vi "Raycaster_CalcObjectDistance.vi"(10 "Location Info":T1, 11 "Decorations In":T5) -> (3 "Decorations Out":T5)   [LabVIEW 2020]
uses:
  Controls/Map_Objects.ctl
  Controls/Map_Object.ctl
  Controls/Map_Position.ctl
  Controls/Game_State.ctl
  Controls/Player_LocationInfo.ctl
  Controls/Player_LocationInfoAxis.ctl
  Globals/FGV_TileVisibleEnum.ctl
  Map_GetMaps.vi
  <vilib>/Utility/file.llb/Application Directory.vi
  <vilib>/rvi/DataTransferAndStorage/Container/XNode/niFpgaContainer.xnode
  <vilib>/rvi/Memory/Memory_Emulation/nirvimemoryFastEmulation.vi
  <vilib>/rvi/Memory/Memory_Emulation/nirvimemoryEmulation.vi
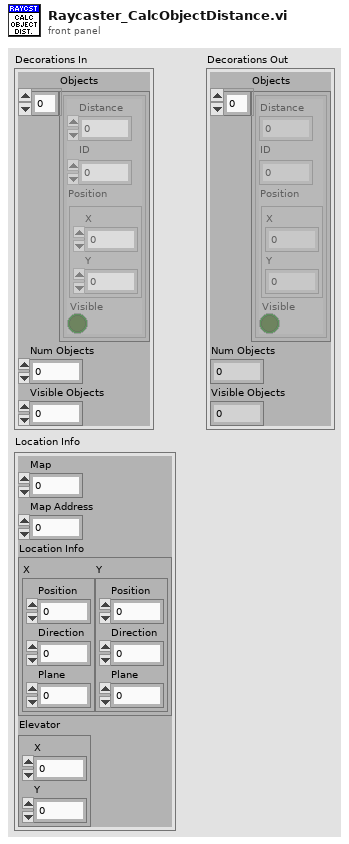
[diagram p1: front panel]
types:
  T1 = typedef "Game_State.ctl" = cluster{"Map":u8, "Map Address":u32, "Location Info":T2, "Elevator":T4}
  T2 = typedef "Player_LocationInfo.ctl" = cluster{"X":T3, "Y":T3}
  T3 = typedef "Player_LocationInfoAxis.ctl" = cluster{"Position":fxp<+/-,32,16>, "Direction":fxp<+/-,32,16>, "Plane":fxp<+/-,32,16>}
  T4 = typedef "Map_Position.ctl" = cluster{"X":fxp<+/-,32,16>, "Y":fxp<+/-,32,16>}
  T5 = typedef "Map_Objects.ctl" = cluster{"Objects":T6[], "Num Objects":i16, "Visible Objects":i16}
  T6 = typedef "Map_Object.ctl" = cluster{"Distance":fxp<+/-,32,16>, "ID":u8, "Position":T4, "Visible":bool}
  T7 = typedef "FGV_TileVisibleEnum.ctl" = enum16{"Reset", "Set Value", "Read Value"}
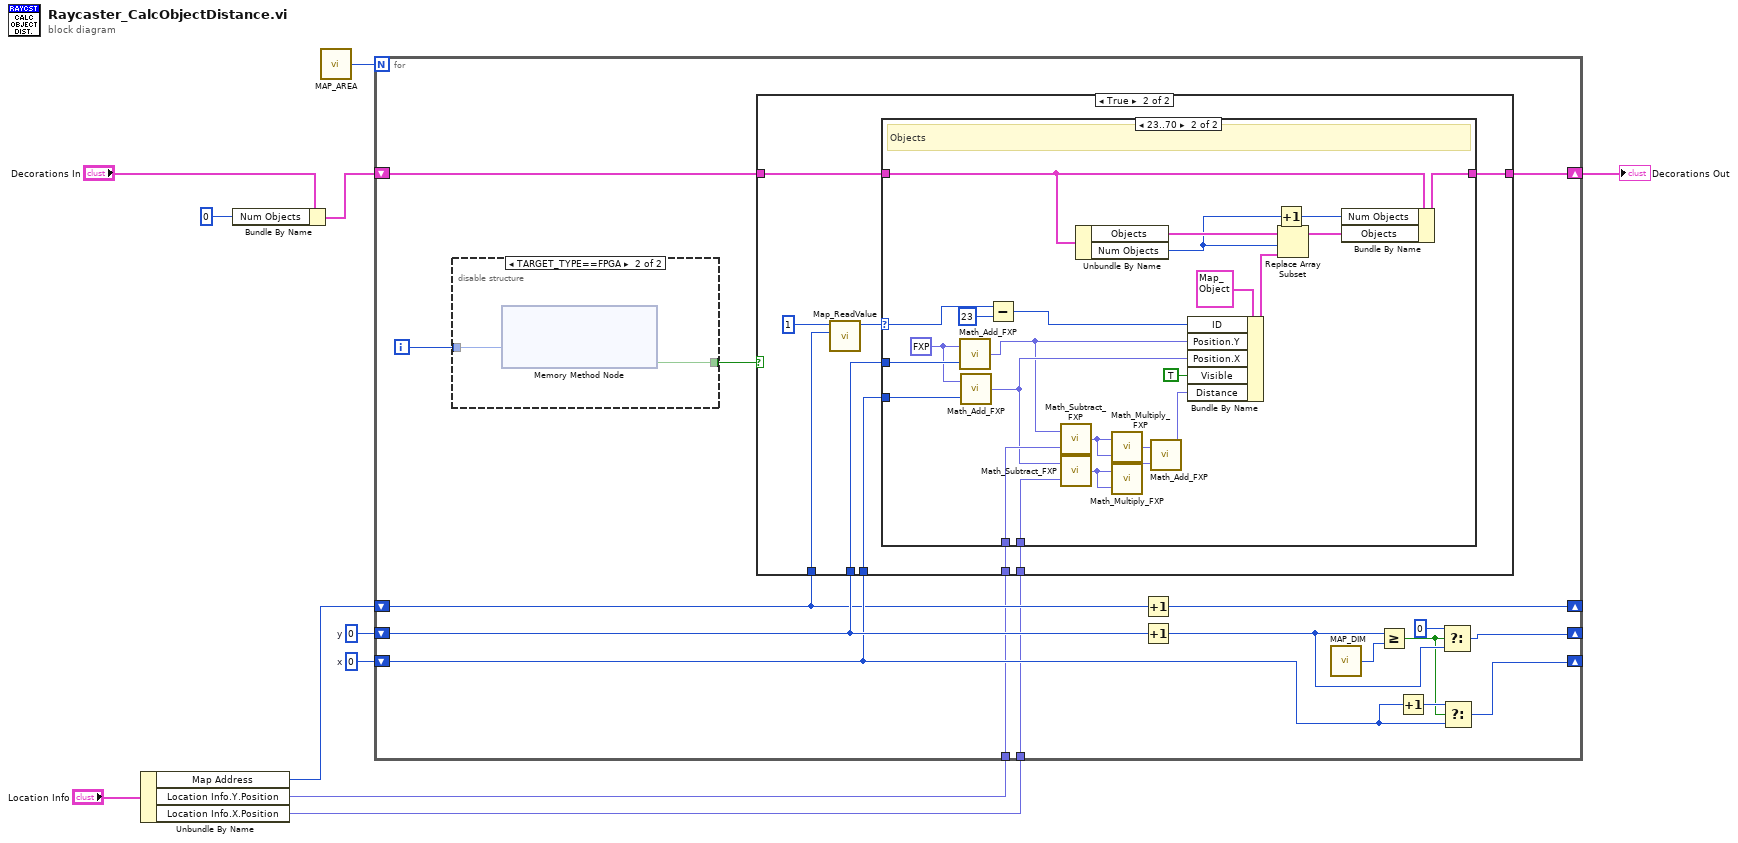
[diagram p0: block diagram]
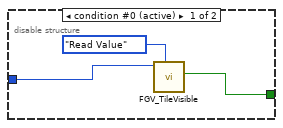
[diagram p4: hidden frame]
diagram:
  w7 = i16 0  # y
  w8 = i16 0  # x
  n1 = Unbundle By Name("Location Info") -> ("Map Address"=w1:u32, "Location Info.Y.Position"=w5:fxp<+/-,32,16>, "Location Info.X.Position"=w4:fxp<+/-,32,16>)
  n2 = Bundle By Name(cluster="Decorations In", "Num Objects"=i16 0 ("Num Decorations")) -> (w3:T5)
  n3 = call "MAP_AREA.vi"() -> ("MAP_DIM"=w6:i16)
  n4 = for {
    N: w6 -> [_]
    shift-right: [w23] -> _
    shift-left: w1 -> [w18]
    shift-right: [w21] -> _
    shift-left: w8 -> [w19]
    shift-right: [w22] -> _
    shift-left: w7 -> [w20]
    shift-right: [w16] -> w10
    shift-left: w3 -> [w17]
    tunnel: w5 -> [w13]
    tunnel: w4 -> [w12]
    i -> [w15]
    n5 = disable-structure shown="TARGET_TYPE==FPGA" {
      disable-tunnel: w15 -> [w64 w67]
      disable-tunnel: [w65 w68] -> w14
      frame condition #0 (active) {
        n6 = call "FGV_TileVisible.vi"("Tile Visible FGV"=FGV_TileVisibleEnum."Read Value", "Index"=w64) -> ("Value Out"=w65:bool)  [unwired: 9 in]
      }
      frame condition #1 {
        n7 = xnode ("Memory Method Node")("Address"=w67) -> ("Data"=w68:bool)  [unwired: 1 in, 1 out]
      }
    }
    n8 = case shown="True" w14 {
      tunnel: w20 -> [_ w36]
      tunnel: w19 -> [_ w35]
      tunnel: w18 -> [_ w34]
      tunnel: w17 -> [w29 w33]
      tunnel: [w29 w32] -> w16
      tunnel: w13 -> [_ w31]
      tunnel: w12 -> [_ w30]
      frame False {
      }
      frame True {
        n9 = call "Map_ReadValue.vi"("Address"=w34, "Plane"=u8 1) -> ("Value"=w37:u8)  [unwired: 9 in]
        n10 = case shown="23..70" w37 {
          selector: w37 -> [_ w56]
          tunnel: w36 -> [_ w55]
          tunnel: w35 -> [_ w54]
          tunnel: w33 -> [w39 w63]
          tunnel: [w39 w60] -> w32
          tunnel: w31 -> [_ w48]
          tunnel: w30 -> [_ w47]
          frame Default {
          }
          frame 23..70 {
            w53 = fxp<+/-,32,16> 0.5 ("x")
            # "Objects"
            n11 = call "Math_Add_FXP.vi"("y"=w55, "x"=w53) -> ("x*y"=w41:fxp<+/-,32,16>)
            n12 = call "Math_Add_FXP.vi"("y"=w54, "x"=w53) -> ("x*y"=w42:fxp<+/-,32,16>)
            n13 = Subtract(x=w56, y=u8 23) -> (x-y=w50:u8)
            n14 = call "Math_Subtract_FXP.vi"("y"=w48, "x"=w41) -> ("x*y"=w43:fxp<+/-,32,16>)
            n15 = call "Math_Subtract_FXP.vi"("y"=w47, "x"=w42) -> ("x*y"=w44:fxp<+/-,32,16>)
            n16 = Unbundle By Name(w63) -> ("Objects"=w61:T6[], "Num Objects"=w59:i16)
            n17 = call "Math_Multiply_FXP.vi"("y"=w43, "x"=w43) -> ("x*y"=w45:fxp<+/-,32,16>)
            n18 = call "Math_Multiply_FXP.vi"("y"=w44, "x"=w44) -> ("x*y"=w46:fxp<+/-,32,16>)
            n19 = call "Math_Add_FXP.vi"("y"=w46, "x"=w45) -> ("x*y"=w40:fxp<+/-,32,16>)
            n20 = Bundle By Name(cluster=T6 {"Distance"=0.0, "ID"=0, "Position"={"X"=0.0, "Y"=0.0}, "Visible"=FALSE} ("new element/subarray"), "ID"=w50, "Position.Y"=w41, "Position.X"=w42, "Visible"=TRUE, "Distance"=w40) -> (w52:T6)
            n21 = Increment(x=w59) -> (x+1=w58:i16)
            n22 = Replace Array Subset(array=w61, new element=w52, index=w59) -> (w62:T6[])
            n23 = Bundle By Name(cluster=w63, "Num Objects"=w58, "Objects"=w62) -> (w60:T5)
          }
        }
      }
    }
    n24 = Increment(x=w18) -> (x+1=w23:u32)
    n25 = Increment(x=w20) -> (x+1=w27:i16)
    n26 = call "MAP_DIM.vi"() -> ("MAP_DIM"=w28:i16)
    n27 = Greater Or Equal?(x=w27, y=w28) -> (x >= y?=w24:bool)
    n28 = Increment(x=w19) -> (x+1=w25:i16)
    n29 = Select(t=i16 0, s=w24, f=w27) -> (s? t:f=w22:i16)
    n30 = Select(t=w25, s=w24, f=w19) -> (s? t:f=w21:i16)
  }
  "Decorations Out" <- w10
